vi "Particle_Enclosing_Circle.vi"() -> ()   [LabVIEW 2017]
panel:
  out "Bounding Box":cluster{dbl, dbl, dbl, dbl}
  out "Center":cluster{i32, i32}
  out "Radius":dbl
  out "Time needed":u32
  out "Image":T1(plugin-control)
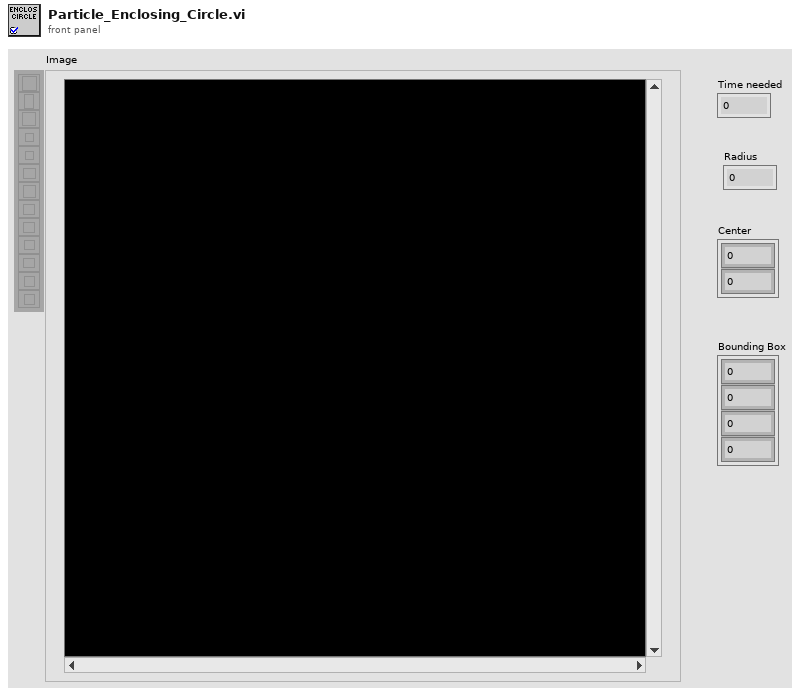
[diagram p1: front panel]
types:
  T1 = typedef "IMAQ Image.ctl" = refnum<image>
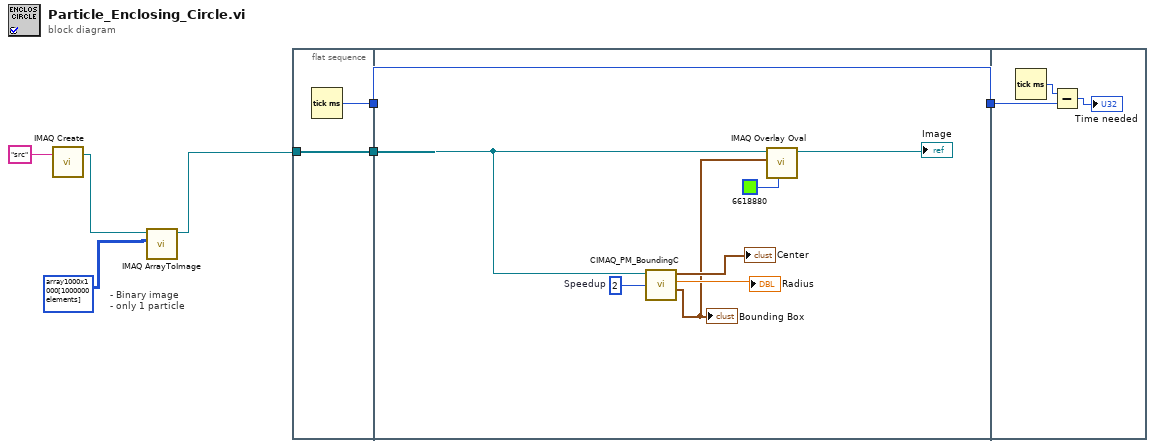
[diagram p0: block diagram]
diagram:
  # "- Binary image \n- only 1 particle"
  n1 = call "IMAQ Create"("Image Name"="src") -> ("New Image"=w1:T1)  [unwired: 4 in, 1 out]
  n2 = call "IMAQ ArrayToImage"("Image Pixels (U8)"=u8[][] array1000x1000[1000000 elements], "Image"=w1) -> ("Image Out"=w3:T1)  [unwired: 8 in, 1 out]
  n3 = flat-sequence {
    tunnel: w3 -> [w9]
    tunnel: [w9] -> w7
    tunnel: [w8] -> w6
    tunnel: w7 -> [w13]
    tunnel: w6 -> [w17]
    tunnel: [w17] -> w5
    tunnel: w5 -> [w19]
    frame #0 {
      n4 = Tick Count (ms)() -> (millisecond timer value=w8:u32)
    }
    frame #1 {
      w16 = 2  # Speedup
      n5 = call "CIMAQ_PM_BoundingC.vi"("Speedup"=w16, "Imag in"=w13) -> ("Bounding Box"=w11:cluster{dbl, dbl, dbl, dbl}, "Radius"=→"Radius":dbl, "Center"=→"Center":cluster{i32, i32})  [unwired: 6 in, 1 out]
      "Bounding Box" <- w11
      n6 = call "IMAQ Overlay Oval"("Color"=u32 6618880, "Bounding Rectangle"=w11, "Image"=w13) -> ("Image Out"=→"Image":T1)  [unwired: 7 in, 1 out]
    }
    frame #2 {
      n7 = Tick Count (ms)() -> (millisecond timer value=w20:u32)
      n8 = Subtract(x=w20, y=w19) -> (x-y=→"Time needed":u32)
    }
  }
